vi "AI Readback.vi"(7 "Box ID":u8=1, 8 "error in (no error)":errorcluster, 10 "Channel":u16=1 min=1 max=8 step=1, 11 "CAN in":refnum<class "XNET_BS120x.lvclass">) -> (0 "error out":errorcluster, 2 "Voltage":dbl, 3 "CAN out":refnum<class "XNET_BS120x.lvclass">)   [LabVIEW 2021, in "BS120x Driver.lvlib" / "XNET_BS120x.lvclass"]
uses:
  XNET_BS120x.lvclass
  BS120x.lvclass
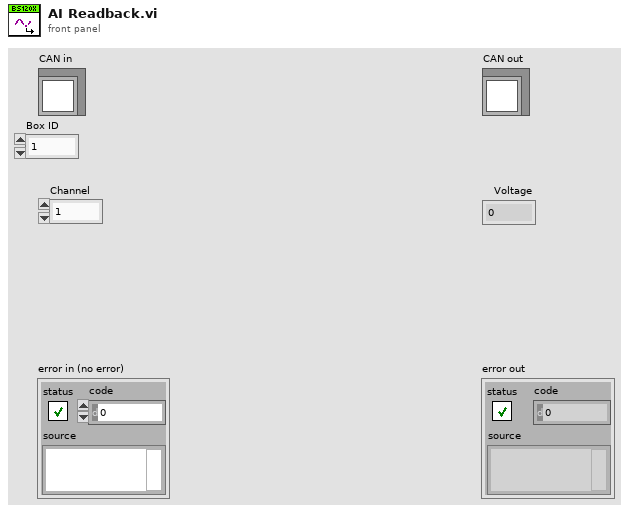
[diagram p1: front panel]
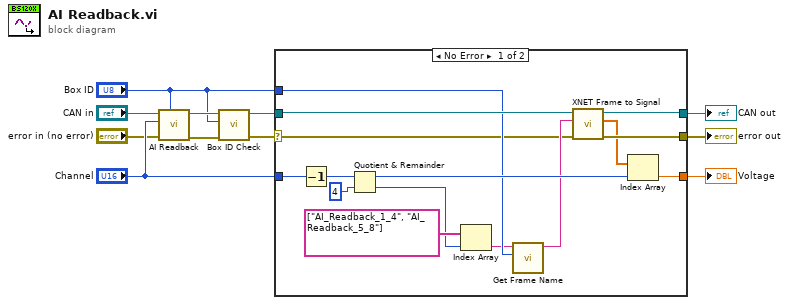
[diagram p0: block diagram]
diagram:
  n1 = call-parent "AI Readback.vi"("Box ID"="Box ID", "error in (no error)"="error in (no error)", "Channel"="Channel", "BS120x in"="CAN in") -> ("error out"=w2:errorcluster, "BS120x out"=w5:refnum<class "XNET_BS120x.lvclass">)  [unwired: 5 in, 1 out]
  n2 = call "Box ID Check.vi"("error in (no error)"=w2, "Box ID"="Box ID", "CAN in"=w5) -> ("error out"=w6:errorcluster, "CAN out"=w7:refnum<class "XNET_BS120x.lvclass">)  [unwired: 7 in]
  n3 = case shown="No Error" w6 {
    selector: w6 -> [w15 w28]
    tunnel: "Channel" -> [w24 _]
    tunnel: w7 -> [w23 w27]
    tunnel: [w22 w27] -> w11
    tunnel: [w21 w28] -> w10
    tunnel: [w18 _] -> w9
    tunnel: "Box ID" -> [w16 _]
    frame No Error {
      n4 = Decrement(x=w24) -> (x-1=w25:u16)
      n5 = Quotient & Remainder(x=w25, y=u16 4) -> (x-y*floor(x/y)=w20:u16, floor(x/y)=w12:u16)
      n6 = Index Array(array=string[] ["AI_Readback_1_4", "AI_Readback_5_8"], index=w12) -> (element=w14:string)
      n7 = call "Get Frame Name.vi"("Box ID"=w16, "Frame Name"=w14) -> ("Frame Name out"=w17:string)  [unwired: 9 in]
      n8 = call "XNET Frame to Signal.vi"("error in (no error)"=w15, "Frame"=w17, "CAN in"=w23) -> ("error out"=w21:errorcluster, "signal data"=w19:dbl[], "CAN out"=w22:refnum<class "XNET_BS120x.lvclass">)  [unwired: 6 in]
      n9 = Index Array(array=w19, index=w20) -> (element=w18:dbl)
    }
    frame Error {
    }
  }
  "error out" <- w10
  "CAN out" <- w11
  "Voltage" <- w9
